vi "StageProcessor.vi"(11 "Microscope in":refnum<class "Microscope.lvclass">) -> ()   [LabVIEW 2012]
uses:
  classes/Microscope.lvclass
  variables/GlobalUI.vi
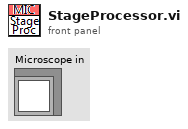
[diagram p1: front panel]
types:
  T1 = typedef "StageEvent.ctl" = enum16{"stage.TimeOut", "stage.FlushData", "stage.GetPosition", "stage.Init", "stage.MoveTo1", "stage.MoveTo2", "stage.MoveTo3", "stage.Stop"}
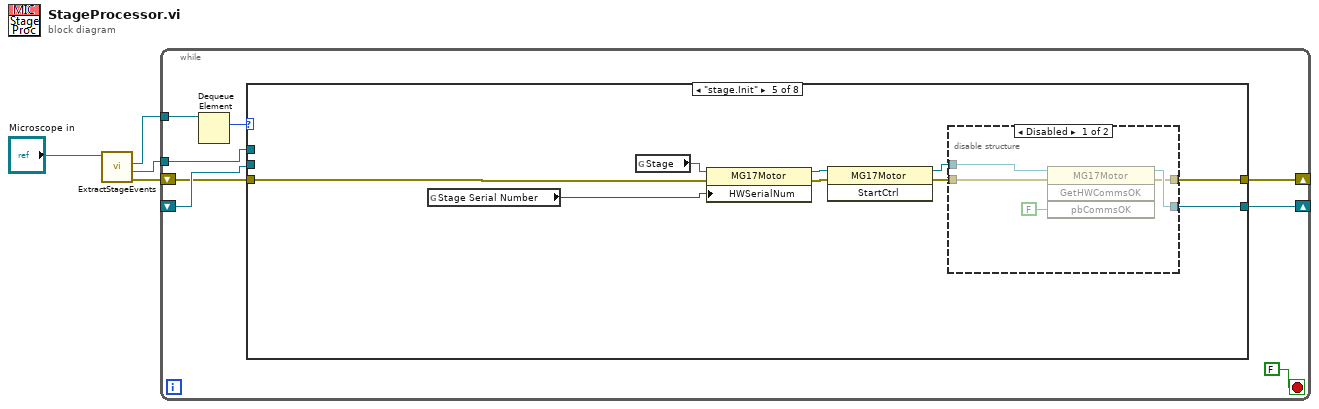
[diagram p0: block diagram]
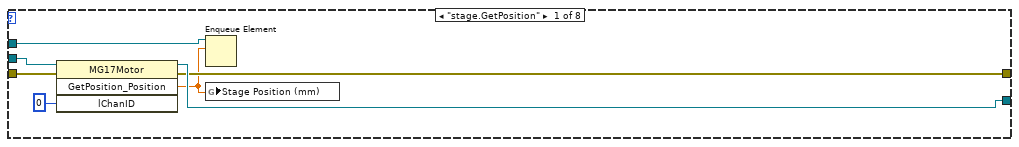
[diagram p2: hidden frame]
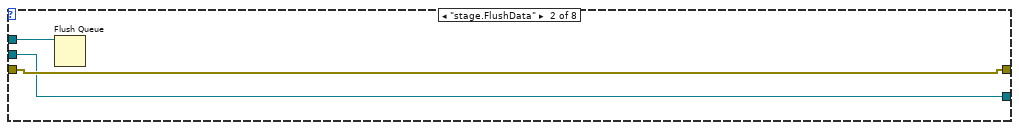
[diagram p3: hidden frame]
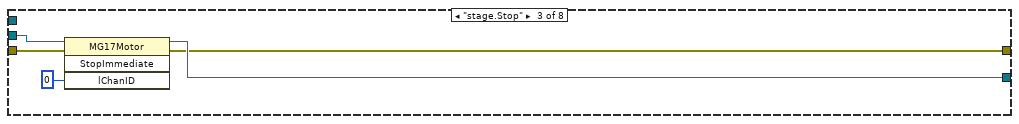
[diagram p4: hidden frame]
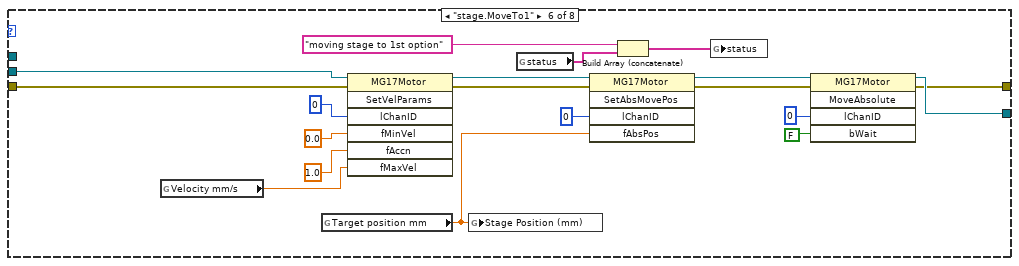
[diagram p7: hidden frame]
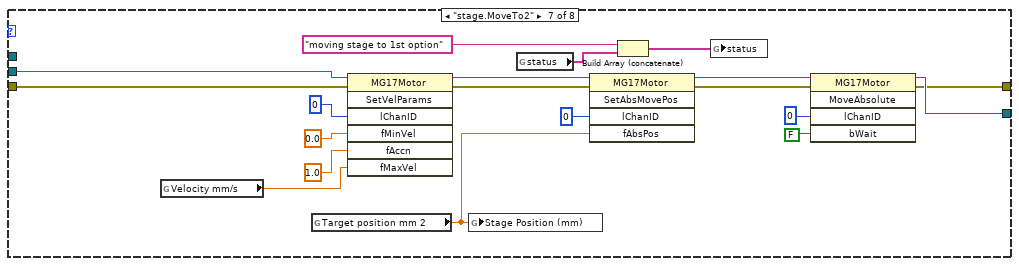
[diagram p8: hidden frame]
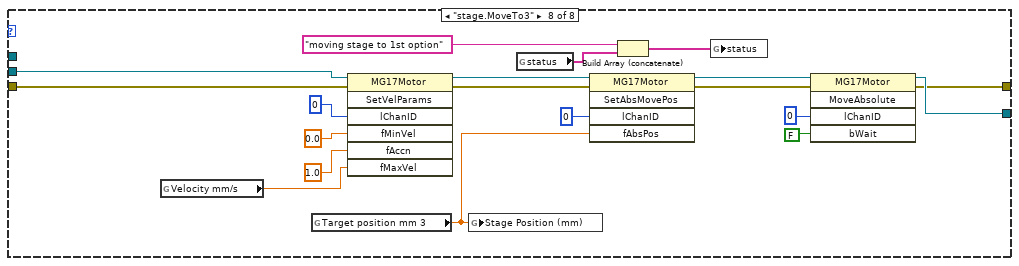
[diagram p9: hidden frame]
diagram:
  n1 = call "ExtractStageEvents.vi"("Microscope in"="Microscope in") -> ("error out"=w2:errorcluster, "X Data"=w1:refnum<queue>, "Stage events"=w3:refnum<queue>)  [unwired: 7 in, 1 out]
  n2 = while {
    tunnel: w3 -> [w10]
    shift-right: [w9] -> _
    shift-left: _ -> [w8]
    shift-right: [w7] -> _
    shift-left: w2 -> [w6]
    tunnel: w1 -> [w5]
    stop <- FALSE stop-if-true
    n3 = Dequeue Element(queue=w10) -> (element=w11:T1)  [unwired: 2 in, 3 out]
    n4 = case shown="\"stage.Init\"" w11 {
      tunnel: [w17 w20 w26 w29 w33 w51 w70 w89] -> w9
      tunnel: w8 -> [w18 w20 w27 w29 _ w52 w71 w90]
      tunnel: w6 -> [w16 w21 w24 w28 w30 w46 w65 w87]
      tunnel: [w15 w21 w25 w28 w32 w49 w66 w84] -> w7
      tunnel: w5 -> [w14 w22 _ _ _ _ _ _]
      frame "stage.GetPosition" {
        n5 = invoke class="MG17Motor" method="GetPosition_Position"(reference=w18, error in=w16, "lChanID"=0) -> (reference out=w17:refnum<k7>, error out=w15:errorcluster, "GetPosition_Position"=w13:sgl)  [unwired: 1 in, 1 out]
        n6 = Enqueue Element(queue=w14, element=w13) -> ()  [unwired: 2 in, 3 out]
        n7 = global write "GlobalUI.vi" "Stage Position (mm)"(w13) -> ()
      }
      frame "stage.FlushData" {
        n8 = Flush Queue(queue=w22) -> ()  [unwired: 1 in, 3 out]
      }
      frame "stage.Stop" {
        n9 = invoke class="MG17Motor" method="StopImmediate"(reference=w27, error in=w24, "lChanID"=0) -> (reference out=w26:refnum<k7>, error out=w25:errorcluster)  [unwired: 1 in, 2 out]
      }
      frame "stage.TimeOut", Default {
      }
      frame "stage.Init" {
        n10 = global read "GlobalUI.vi" "Stage Serial Number"() -> (w34:i32)
        n11 = global read "GlobalUI.vi" "Stage"() -> (w35:refnum<k7>)
        n12 = property class="MG17Motor"(reference=w35, error in=w30, "HWSerialNum"=w34) -> (reference out=w36:refnum<k7>, error out=w31:errorcluster)
        n13 = invoke class="MG17Motor" method="StartCtrl"(reference=w36, error in=w31) -> (reference out=w38:refnum<k7>, error out=w37:errorcluster)  [unwired: 1 in, 1 out]
        n14 = disable-structure shown="Disabled" {
          disable-tunnel: w38 -> [w43 w45]
          disable-tunnel: w37 -> [w42 w44]
          disable-tunnel: [w40 w45] -> w33
          disable-tunnel: [w39 w44] -> w32
          frame Disabled {
            n15 = invoke class="MG17Motor" method="GetHWCommsOK"(reference=w43, error in=w42, "pbCommsOK"=FALSE) -> (reference out=w40:refnum<k7>, error out=w39:errorcluster)  [unwired: 1 in, 2 out]
          }
          frame Enabled {
          }
        }
      }
      frame "stage.MoveTo1" {
        n16 = global read "GlobalUI.vi" "Velocity mm/s"() -> (w53:sgl)
        n17 = global read "GlobalUI.vi" "Target position mm"() -> (w54:dbl)
        n18 = invoke class="MG17Motor" method="SetVelParams"(reference=w52, error in=w46, "lChanID"=0, "fMinVel"=sgl 0.0, "fAccn"=sgl 1.0, "fMaxVel"=w53) -> (reference out=w58:refnum<k7>, error out=w47:errorcluster)  [unwired: 1 in, 5 out]
        n19 = global write "GlobalUI.vi" "Stage Position (mm)"(w54) -> ()
        n20 = global read "GlobalUI.vi" "status"() -> (w64:string[])
        n21 = invoke class="MG17Motor" method="SetAbsMovePos"(reference=w58, error in=w47, "lChanID"=0, "fAbsPos"=w54) -> (reference out=w59:refnum<k7>, error out=w48:errorcluster)  [unwired: 1 in, 3 out]
        n22 = Build Array (concatenate)("moving stage to 1st option" ("status"), w64) -> (w63:string[])
        n23 = global write "GlobalUI.vi" "status"(w63) -> ()
        n24 = invoke class="MG17Motor" method="MoveAbsolute"(reference=w59, error in=w48, "lChanID"=0, "bWait"=FALSE) -> (reference out=w51:refnum<k7>, error out=w49:errorcluster)  [unwired: 1 in, 3 out]
      }
      frame "stage.MoveTo2" {
        n25 = global read "GlobalUI.vi" "Velocity mm/s"() -> (w72:sgl)
        n26 = global read "GlobalUI.vi" "Target position mm 2"() -> (w73:dbl)
        n27 = invoke class="MG17Motor" method="SetVelParams"(reference=w71, error in=w65, "lChanID"=0, "fMinVel"=sgl 0.0, "fAccn"=sgl 1.0, "fMaxVel"=w72) -> (reference out=w77:refnum<k7>, error out=w68:errorcluster)  [unwired: 1 in, 5 out]
        n28 = global write "GlobalUI.vi" "Stage Position (mm)"(w73) -> ()
        n29 = global read "GlobalUI.vi" "status"() -> (w83:string[])
        n30 = invoke class="MG17Motor" method="SetAbsMovePos"(reference=w77, error in=w68, "lChanID"=0, "fAbsPos"=w73) -> (reference out=w78:refnum<k7>, error out=w67:errorcluster)  [unwired: 1 in, 3 out]
        n31 = Build Array (concatenate)("moving stage to 1st option" ("status"), w83) -> (w82:string[])
        n32 = global write "GlobalUI.vi" "status"(w82) -> ()
        n33 = invoke class="MG17Motor" method="MoveAbsolute"(reference=w78, error in=w67, "lChanID"=0, "bWait"=FALSE) -> (reference out=w70:refnum<k7>, error out=w66:errorcluster)  [unwired: 1 in, 3 out]
      }
      frame "stage.MoveTo3" {
        n34 = global read "GlobalUI.vi" "Velocity mm/s"() -> (w91:sgl)
        n35 = global read "GlobalUI.vi" "Target position mm 3"() -> (w92:dbl)
        n36 = invoke class="MG17Motor" method="SetVelParams"(reference=w90, error in=w87, "lChanID"=0, "fMinVel"=sgl 0.0, "fAccn"=sgl 1.0, "fMaxVel"=w91) -> (reference out=w96:refnum<k7>, error out=w86:errorcluster)  [unwired: 1 in, 5 out]
        n37 = global write "GlobalUI.vi" "Stage Position (mm)"(w92) -> ()
        n38 = global read "GlobalUI.vi" "status"() -> (w102:string[])
        n39 = invoke class="MG17Motor" method="SetAbsMovePos"(reference=w96, error in=w86, "lChanID"=0, "fAbsPos"=w92) -> (reference out=w97:refnum<k7>, error out=w85:errorcluster)  [unwired: 1 in, 3 out]
        n40 = Build Array (concatenate)("moving stage to 1st option" ("status"), w102) -> (w101:string[])
        n41 = global write "GlobalUI.vi" "status"(w101) -> ()
        n42 = invoke class="MG17Motor" method="MoveAbsolute"(reference=w97, error in=w85, "lChanID"=0, "bWait"=FALSE) -> (reference out=w89:refnum<k7>, error out=w84:errorcluster)  [unwired: 1 in, 3 out]
      }
    }
  }
